vi "DRAFT1.vi"() -> ()   [LabVIEW 2021]
uses:
  <vilib>/Analysis/3filter.llb/Butterworth Filter (DBL).vi
  <vilib>/Analysis/NI_AALBase.lvlib
  <vilib>/ptbypt/NI_PtbyPt.lvlib
panel:
  out "Array Size":u32
  out "Elapsed time in ms":u32
  in  "stop":bool
  in  "error in (no error)":errorcluster
  out "error out":errorcluster
  in  "loop 1":i32
  out "Waveform Graph 6":dynamicdata(graph)
  out "Waveform Graph 5":dynamicdata(graph)
  out "Waveform Graph 4":dynamicdata(graph)
  out "Waveform Graph 3":dbl[](graph)
  out "Waveform Graph 2":dynamicdata(graph)
  out "Array":dbl[](array[numeric])
  in  "Boolean":bool
  out "Waveform Graph":dbl[](graph)
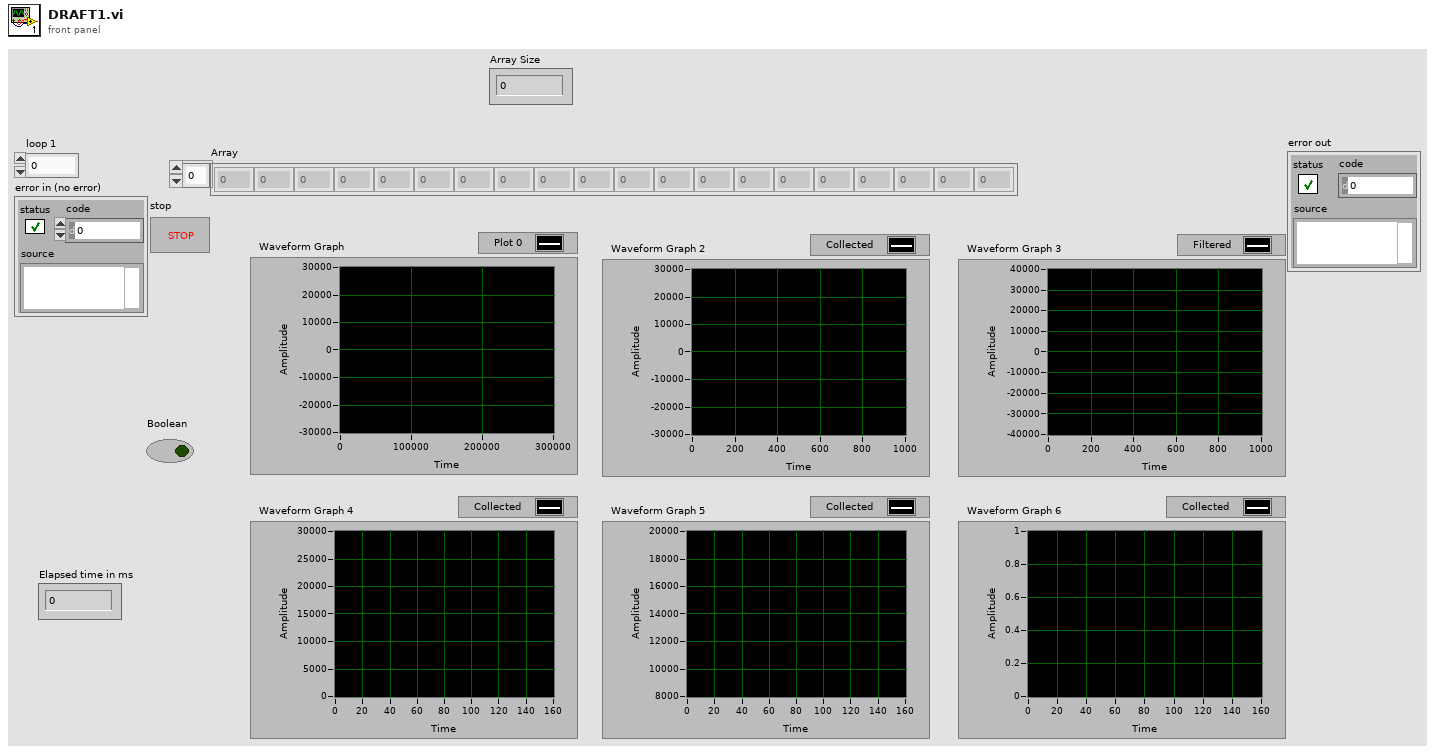
[diagram p1: front panel]
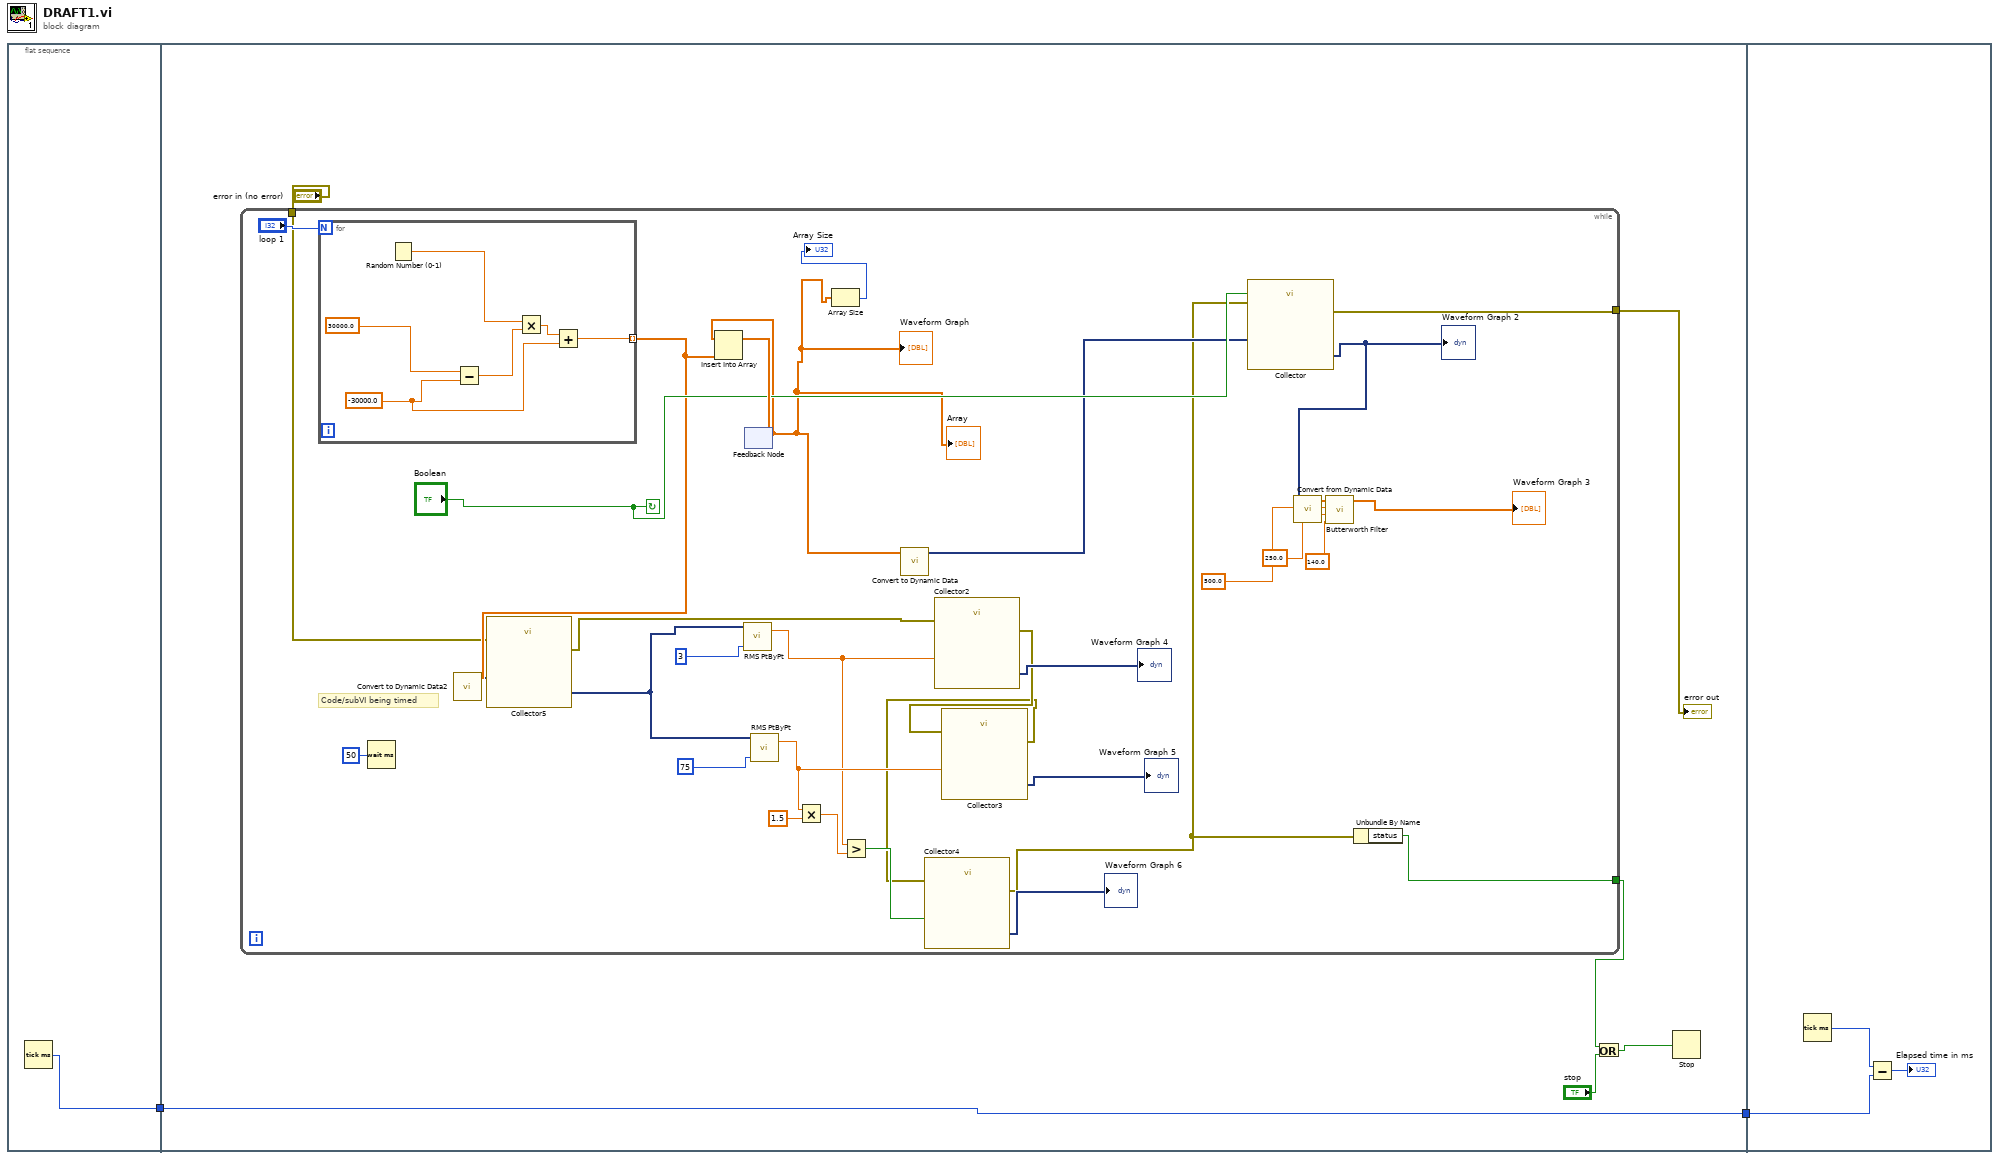
[diagram p0: block diagram]
diagram:
  n1 = flat-sequence {
    tunnel: [w3] -> w2
    tunnel: [w10] -> w1
    tunnel: w2 -> [w10]
    tunnel: w1 -> [w49]
    frame #0 {
      n2 = Tick Count (ms)() -> (millisecond timer value=w3:u32)
    }
    frame #1 {
      # "Code/subVI being timed"
      n3 = while {
        tunnel: "error in (no error)" -> [w19]
        tunnel: [w15] -> w7
        tunnel: [w13] -> w6
        stop <- "Boolean" continue-if-true
        n4 = for {
          N: "loop 1" -> [_]
          tunnel: [w43] -> w22 mode=indexing
          w45 = -30000.0 ("y")
          n5 = Random Number (0-1)() -> (number: 0 to 1=w44:dbl)
          n6 = Subtract(x=30000.0, y=w45) -> (x-y=w48:dbl)
          n7 = Multiply(x=w44, y=w48) -> (x*y=w47:dbl)
          n8 = Add(x=w47, y=w45) -> (x+y=w43:dbl)
        }
        n9 = call "Convert to Dynamic Data2"("Array"=w22) -> ("Dynamic Data Type"=w21:dynamicdata)  [unwired: 3 in]
        n10 = call "Collector5"("error in (no error)"=w19, "Signals"=w21) -> ("error out"=w18:errorcluster, "Collected Signals"=w20:dynamicdata)  [unwired: 8 in]
        n11 = call <vilib>:"RMS PtByPt.vi"("sample length"=3, "x"=w20) -> ("rms value"=w26:dbl)  [unwired: 2 in, 1 out]
        n12 = feedback #1() -> (w11:dbl[])  [unwired: 1 in]
        "Array" <- w11
        "Waveform Graph" <- w11
        n13 = Insert Into Array(array=w11, new element=w22) -> (w42:dbl[])  [unwired: 1 in]
        n14 = feedback-in #1(w42) -> ()
        n15 = call <vilib>:"RMS PtByPt.vi"("sample length"=75, "x"=w20) -> ("rms value"=w29:dbl)  [unwired: 2 in, 1 out]
        n16 = Multiply(x=w29, y=1.5) -> (x*y=w27:dbl)
        n17 = Array Size(array=w11) -> (size(s)=→"Array Size":i32)
        n18 = Greater?(x=w26, y=w27) -> (0:w25:bool)
        n19 = call "Convert to Dynamic Data"("Array"=w11) -> ("Dynamic Data Type"=w32:dynamicdata)  [unwired: 3 in]
        n20 = call "Collector2"("error in (no error)"=w18, "Signals"=w26) -> ("error out"=w17:errorcluster, "Collected Signals"=→"Waveform Graph 4":dynamicdata)  [unwired: 8 in]
        n21 = call "Collector3"("error in (no error)"=w17, "Signals"=w29) -> ("error out"=w16:errorcluster, "Collected Signals"=→"Waveform Graph 5":dynamicdata)  [unwired: 8 in]
        n22 = call "Collector4"("error in (no error)"=w16, "Signals"=w25) -> ("error out"=w14:errorcluster, "Collected Signals"=→"Waveform Graph 6":dynamicdata)  [unwired: 8 in]
        n23 = call "Collector"("error in (no error)"=w14, "Enable"="Boolean", "Signals"=w32) -> ("error out"=w15:errorcluster, "Collected Signals"=w35:dynamicdata)  [unwired: 7 in]
        "Waveform Graph 2" <- w35
        n24 = call "Convert from Dynamic Data"("Dynamic Data Type"=w35) -> ("Array"=w37:dbl[])  [unwired: 3 in]
        n25 = call-poly <vilib>:"Butterworth Filter.vi"("low cutoff freq: fl"=140.0, "high cutoff freq: fh"=250.0, "sampling freq: fs"=500.0, "X"=w37) -> ("Filtered X"=→"Waveform Graph 3":dbl[])  [unwired: 4 in, 1 out]
        n26 = Unbundle By Name(w14) -> ("status"=w13:bool)
      }
      "error out" <- w7
      n27 = Wait (ms)(milliseconds to wait=u32 50) -> ()  [unwired: 1 out]
      n28 = Or(x=w6, y="stop") -> (x .or. y?=w4:bool)
      n29 = Stop(stop? (T)=w4) -> ()
    }
    frame #2 {
      n30 = Tick Count (ms)() -> (millisecond timer value=w51:u32)
      n31 = Subtract(x=w51, y=w49) -> (x-y=→"Elapsed time in ms":u32)
    }
  }
